vi "Settings.vi"() -> ()   [LabVIEW 2010]
panel:
  in  "ClusterNameDevices":T1={"Commutator34980A"="34980", "Multimetr34410A"="34410"}
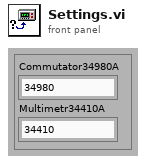
[diagram p1: front panel]
types:
  T1 = cluster{"Commutator34980A":string, "Multimetr34410A":string}
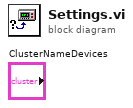
[diagram p0: block diagram]
diagram:
